vi "PID.vi"(8 "Boolean":bool, 11 "Numeric in":dbl) -> (3 "Numeric out":dbl)   [LabVIEW 2017]
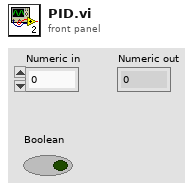
[diagram p1: front panel]
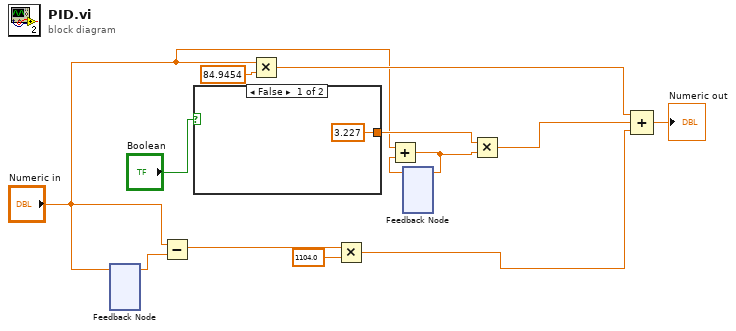
[diagram p0: block diagram]
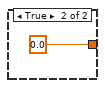
[diagram p2: hidden frame]
diagram:
  n1 = feedback #1() -> (w13:dbl)  [unwired: 1 in]
  n2 = feedback-in #1("Numeric in") -> ()
  n3 = Subtract(x="Numeric in", y=w13) -> (x-y=w9:dbl)
  n4 = case shown="False" "Boolean" {
    tunnel: [3.227 ("x") 0.0 ("x")] -> w2
    frame False {
    }
    frame True {
    }
  }
  n5 = Multiply(x="Numeric in", y=84.9454) -> (x*y=w11:dbl)
  n6 = Multiply(x=w9, y=1104.0) -> (x*y=w8:dbl)
  n7 = feedback #2() -> (w5:dbl)  [unwired: 1 in]
  n8 = Add(x="Numeric in", y=w5) -> (x+y=w6:dbl)
  n9 = feedback-in #2(w6) -> ()
  n10 = Multiply(x=w2, y=w6) -> (x*y=w4:dbl)
  n11 = Compound Arithmetic op=ADD(w11, w4, w8) -> (→"Numeric out":dbl)
